vi "Calib_Analyse_fit.vi"(0 "Calib file":path, 1 "Input points":dbl[][](array[numeric]) format="%.2f", 2 "polynomial order":i32=2, 5 "Fixed n":bool=TRUE, 7 "n":dbl=0.45 format="%.2f", 9 "Point selector 3":cluster{"Y":dbl, "X":dbl, "t/f":bool}[](array[cluster]) {"X" format="%.2f"; "Y" format="%.2f"}, 11 "Point selector 4":T1(array[cluster])=[{"Y"=3.5155385742, "Y2"=3.2773117676, "X"=-15.0, "t/f"=FALSE}, {"Y"=3.4946367187, "Y2"=3.3075422363, "X"=-10.0, "t/f"=FALSE}, {"Y"=3.473232666, "Y2"=3.3353713379, "X"=-5.0, "t/f"=FALSE}, {"Y"=3.454592041, "Y2"=3.3658986816, "X"=0.0, "t/f"=FALSE}, {"Y"=3.4246572266, "Y2"=3.3874455566, "X"=5.0, "t/f"=FALSE}, {"Y"=3.398965332, "Y2"=3.4137351074, "X"=10.0, "t/f"=FALSE}, {"Y"=3.362712646484375, "Y2"=3.428485595703125, "X"=15.0, "t/f"=FALSE}] {"Y2" format="%.2f"; "X" format="%.2f"; "Y" format="%.2f"}) -> (4 "Calib const":string[][](array[string])=[["n", "0.405000"], ["A", "7.730378"], ["B", "6.204067"], ["Av % err", "0.204301"]], 6 "Calibration plot":cluster{cluster{dbl, dbl}[]}[](graph)=[{[{0.8450215822560672, 12.972948762710196}, {0.9063644870167936, 13.35352428024258}, {1.0129933166229186, 14.015056729178777}, {1.0924501688964157, 14.50801239851709}, {1.2215481063301497, 15.308944707524116}, {1.3521910897315237, 16.119462585897956}, {1.4772434835777744, 16.895296069694275}]}, {[{0.8450215822560672, 12.97084622363197}, {0.9063644870167936, 13.353228276297402}, {1.0129933166229186, 14.026771757587431}, {1.0924501688964157, 14.499243467101884}, {1.2215481063301497, 15.307992219000921}, {1.3521910897315237, 16.116882250583185}, {1.4772434835777744, 16.898281339562185}]}], 8 "Average Temp":dbl=19.0 format="%.2f", 10 "Point selector 3 out":cluster{"Y":dbl, "X":dbl, "t/f":bool}[](array[cluster]) {"X" format="%.2f"; "Y" format="%.2f"}, 14 "Coefficients":dbl[][](array[numeric]) format="%.2f", 15 "Point selector 4 out":T1(array[cluster])=[{"Y"=3.5155385742, "Y2"=3.2773117676, "X"=-15.0, "t/f"=FALSE}, {"Y"=3.4946367187, "Y2"=3.3075422363, "X"=-10.0, "t/f"=FALSE}, {"Y"=3.473232666, "Y2"=3.3353713379, "X"=-5.0, "t/f"=FALSE}, {"Y"=3.454592041, "Y2"=3.3658986816, "X"=0.0, "t/f"=FALSE}, {"Y"=3.4246572266, "Y2"=3.3874455566, "X"=5.0, "t/f"=FALSE}, {"Y"=3.398965332, "Y2"=3.4137351074, "X"=10.0, "t/f"=FALSE}, {"Y"=3.362712646484375, "Y2"=3.428485595703125, "X"=15.0, "t/f"=FALSE}] {"Y2" format="%.2f"; "X" format="%.2f"; "Y" format="%.2f"})   [LabVIEW 2014]
uses:
  <vilib>/Analysis/baseanly.llb/Mean (DBL).vi
  Globals/Calib_global.vi
  Acquisition/PWA/PWAtasksGLOBAL.vi
  <vilib>/Analysis/NI_AALBase.lvlib
panel:
  out "GMU:Source:ppm/%Density":dbl format="%.2f"
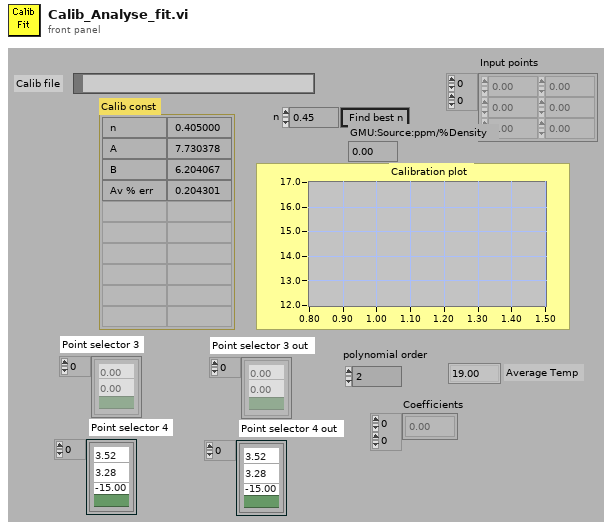
[diagram p1: front panel]
types:
  T1 = cluster{"Y":dbl, "Y2":dbl, "X":dbl, "t/f":bool}[]
  T2 = typedef "Cal_Inst_type.ctl" = enum16{"Propeller anemometer", "Pressure Transducer", "Hot wire", "Cross wire velocity", "Cross wire angle", "Generic Linear", "Generic Polynomial", "Generic BackPoly", "Fast FID", "Thermocouple", "Cold wire", "Pulsed Wire"}
  T3 = cluster{"Y":dbl, "Y":dbl, "X":dbl, "switch":bool}
  T4 = typedef "Ref_Inst_type.ctl" = enum16{"Propellor anemometer", "Pressure Transducer", "Raw voltage", "Pitot-static tube", "Preston tube", "Generic Linear", "Generic Polynomial", "Thermocouple", "LDA", "Enter Value", "ADAM Channel"}
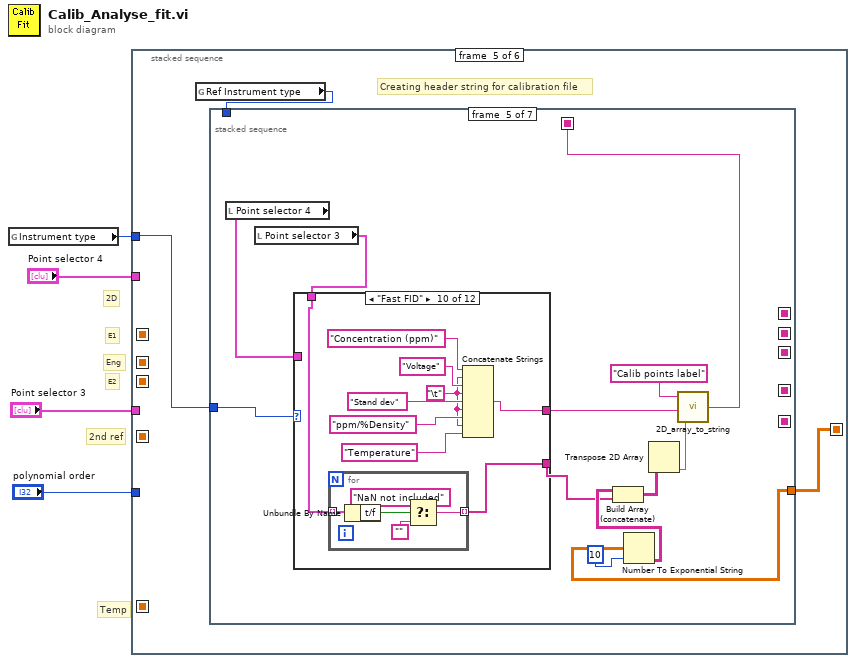
[diagram p0: block diagram]
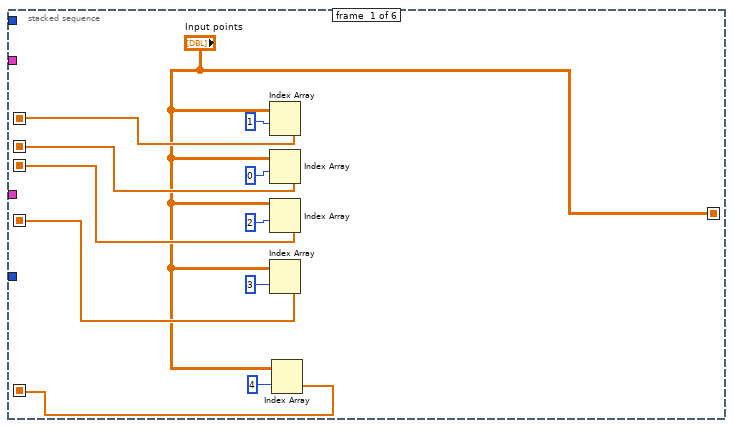
[diagram p2: hidden frame]
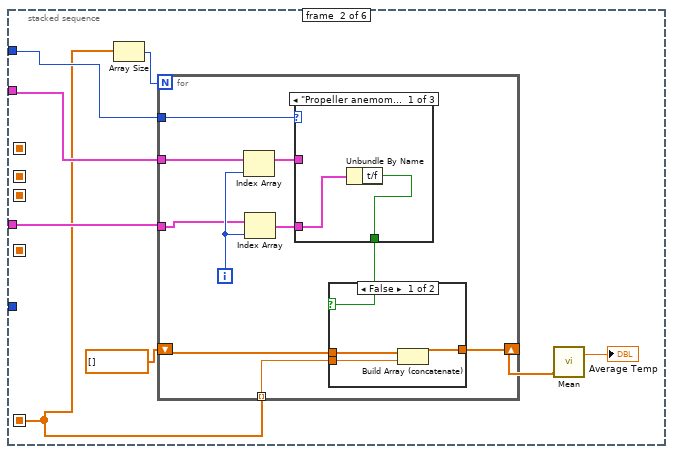
[diagram p3: hidden frame]
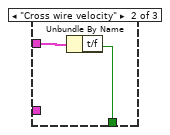
[diagram p5: hidden frame]
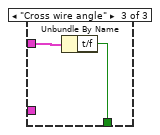
[diagram p6: hidden frame]
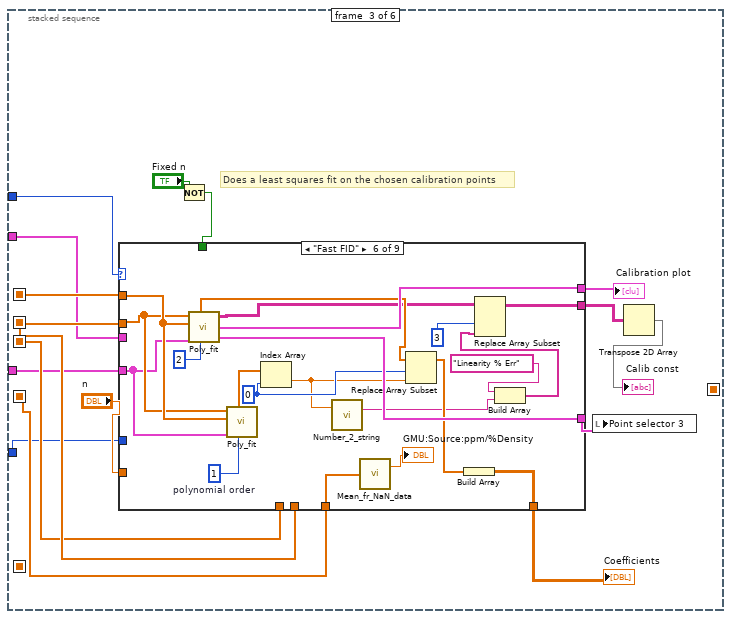
[diagram p7: hidden frame]
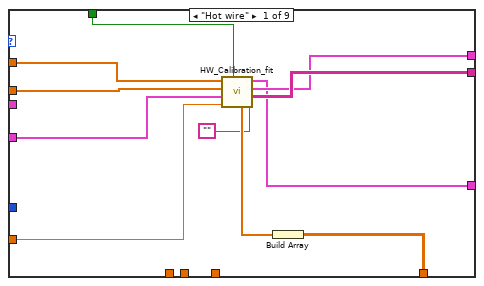
[diagram p8: hidden frame]
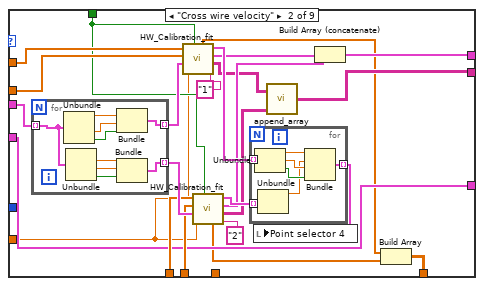
[diagram p9: hidden frame]
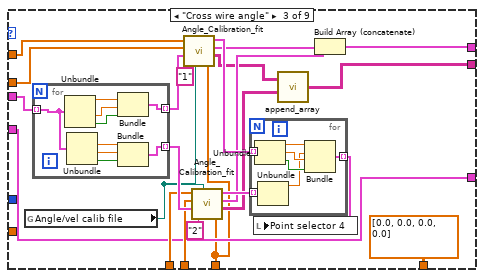
[diagram p10: hidden frame]
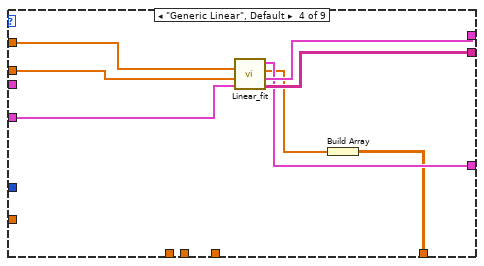
[diagram p11: hidden frame]
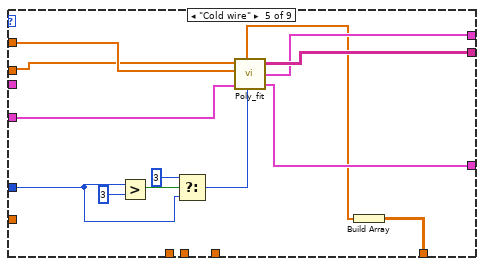
[diagram p12: hidden frame]
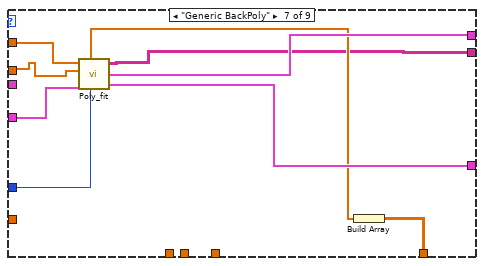
[diagram p13: hidden frame]
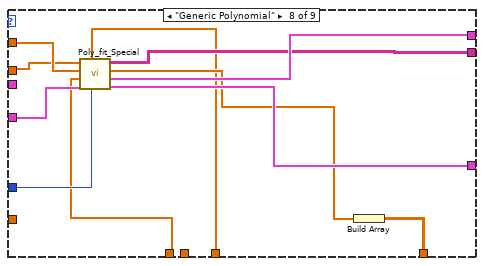
[diagram p14: hidden frame]
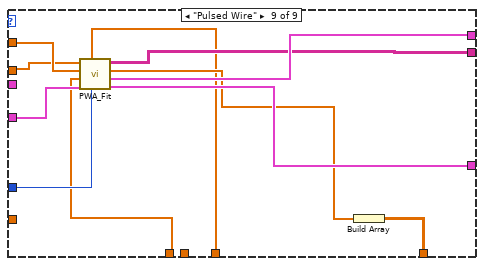
[diagram p15: hidden frame]
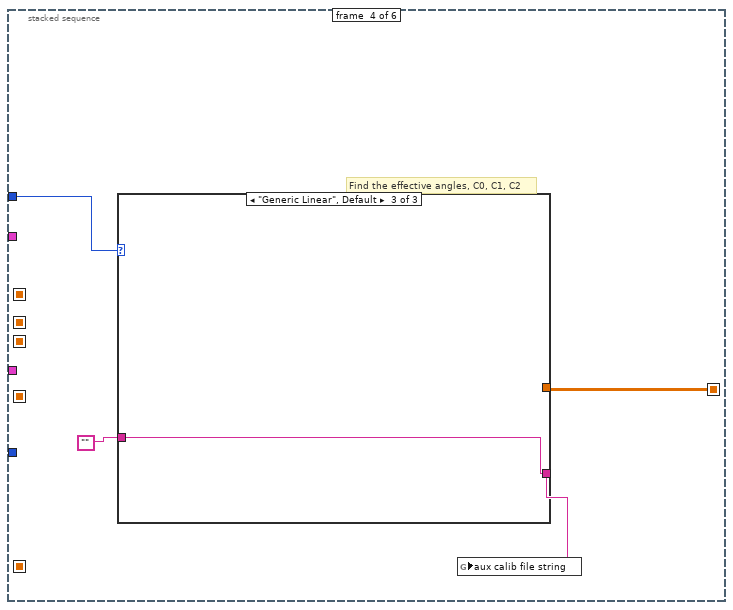
[diagram p16: hidden frame]
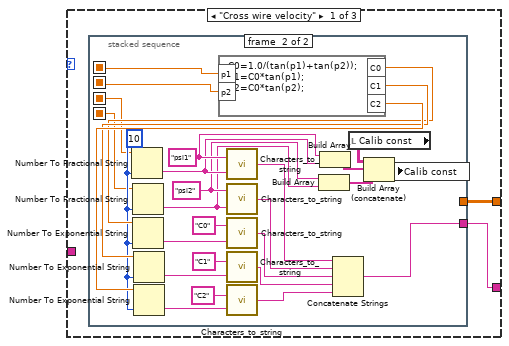
[diagram p17: hidden frame]
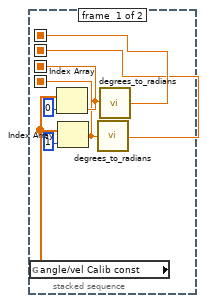
[diagram p18: hidden frame]
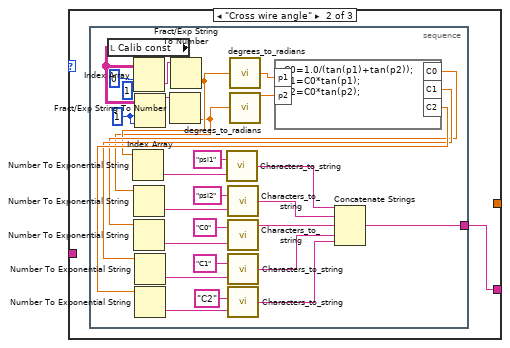
[diagram p19: hidden frame]
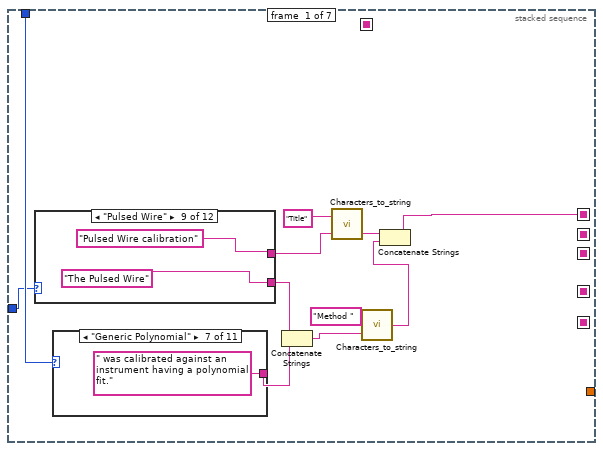
[diagram p20: hidden frame]
diagram:
  # "Temp"
  # "2D"
  # "2nd ref"
  # "E2"
  # "E1"
  # "Eng"
  n1 = global read "Calib_global.vi" "Instrument type"() -> (w4:T2)
  n2 = stacked-sequence {
    seq-local: ["Input points" _ _ _ _ _] -> [_ _ _ w223 w295 _]
    seq-local: [w11 _ _ _ _ _] -> [_ _ w52 _ _ _]
    seq-local: [w10 _ _ _ _ _] -> [_ _ w51 _ _ _]
    seq-local: [w9 _ _ _ _ _] -> [_ _ w50 _ _ _]
    seq-local: [w8 _ _ _ _ _] -> [_ _ w49 _ _ _]
    seq-local: [w5 _ _ _ _ _] -> [_ w17 _ _ _ _]
    tunnel: w4 -> [_ w23 w46 w222 w294 _]
    tunnel: "Point selector 3" -> [_ w22 w48 _ _ _]
    tunnel: "Point selector 4" -> [_ w21 w47 _ _ _]
    tunnel: "polynomial order" -> [_ _ w44 _ _ _]
    frame #0 {
      n3 = Index Array(array="Input points", index (row)=1) -> (element=w11:dbl[])  [unwired: 1 in]
      n4 = Index Array(array="Input points", index (row)=0) -> (element=w10:dbl[])  [unwired: 1 in]
      n5 = Index Array(array="Input points", index (row)=2) -> (element=w9:dbl[])  [unwired: 1 in]
      n6 = Index Array(array="Input points", index (row)=3) -> (element=w8:dbl[])  [unwired: 1 in]
      n7 = Index Array(array="Input points", index (row)=4) -> (element=w5:dbl[])  [unwired: 1 in]
    }
    frame #1 {
      n8 = Array Size(array=w17) -> (size(s)=w16:i32)
      n9 = for {
        N: w16 -> [_]
        tunnel: w23 -> [w33]
        tunnel: w22 -> [w25]
        tunnel: w21 -> [w27]
        shift-right: [w30] -> w18
        shift-left: dbl[] [] -> [w31]
        tunnel: w17 -> [w29] mode=indexing
        i -> [w26]
        n10 = Index Array(array=w27, index=w26) -> (element=w28:cluster{"Y":dbl, "Y2":dbl, "X":dbl, "t/f":bool})
        n11 = Index Array(array=w25, index=w26) -> (element=w24:cluster{"Y":dbl, "X":dbl, "t/f":bool})
        n12 = case shown="\"Propeller anemometer\", Default" w33 {
          tunnel: w24 -> [w39 _ _]
          tunnel: w28 -> [_ w41 w43]
          tunnel: [w38 w40 w42] -> w32
          frame "Propeller anemometer", Default {
            n13 = Unbundle By Name(w39) -> ("t/f"=w38:bool)
          }
          frame "Cross wire velocity" {
            n14 = Unbundle By Name(w41) -> ("t/f"=w40:bool)
          }
          frame "Cross wire angle" {
            n15 = Unbundle By Name(w43) -> ("t/f"=w42:bool)
          }
        }
        n16 = case shown="False" w32 {
          tunnel: w31 -> [w36 w37]
          tunnel: [w35 w37] -> w30
          tunnel: w29 -> [w34 _]
          frame False {
            n17 = Build Array (concatenate)(w36, w34) -> (w35:dbl[])
          }
          frame True {
          }
        }
      }
      n18 = call-poly <vilib>:"Mean.vi"("X"=w18) -> ("mean"=→"Average Temp":dbl)  [unwired: 1 out]
    }
    frame #2 {
      # "Does a least squares fit on the chosen calibration points"
      n19 = Not(x="Fixed n") -> (.not. x?=w54:bool)
      n20 = case shown="\"Fast FID\"" w46 {
        tunnel: [w65 w82 w120 w151 w166 w189 w198 w209 w220] -> w57
        tunnel: w52 -> [w70 w94 w132 w156 w165 w178 w195 w207 w218]
        tunnel: w51 -> [w69 w93 w131 w155 w164 w177 w194 w206 w217]
        tunnel: w54 -> [w68 w80 _ _ _ _ _ _ _]
        tunnel: w47 -> [_ w83 w121 _ _ _ _ _ _]
        tunnel: [w67 w76 w114 w154 w169 w179 w192 w203 w214] -> w55
        tunnel: [w66 w84 w122 w153 w168 w190 w199 w210 w221] -> w56
        tunnel: w51 -> [_ w89 w127 _ _ _ _ _ _]
        tunnel: w50 -> [_ w88 w126 _ _ _ _ w201 w212]
        tunnel: w48 -> [w64 w82 w120 w152 w167 w176 w196 w205 w216]
        tunnel: "n" -> [w63 w79 _ _ _ _ _ _ _]
        tunnel: w49 -> [_ _ w113 _ _ w171 _ w200 w211]
        tunnel: [w61 w73 dbl[][] [[0.0, 0.0], [0.0, 0.0]] w149 w158 w188 w197 w208 w219] -> w45
        tunnel: w44 -> [_ _ _ _ w157 _ w191 w202 w213]
        frame "Hot wire" {
          n21 = call "HW_Calibration_fit.vi"("coeff suffix"="", "Fixed n (F)"=w68, "n input  (0.45)"=w63, "Point selector"=w64, "Velocity"=w69, "HW voltage"=w70) -> ("Calib const"=w67:string[][], "Calibration plot"=w66:cluster{cluster{dbl, "mse":dbl}[]}[], "Point selector"=w65:cluster{"Y":dbl, "X":dbl, "switch":bool}[], "Coefficients"=w62:dbl[])
          n22 = Build Array(w62) -> (w61:dbl[][])
        }
        frame "Cross wire velocity" {
          n23 = for {
            tunnel: w83 -> [w106] mode=indexing
            tunnel: [w107] -> w92 mode=indexing
            tunnel: [w105] -> w90 mode=indexing
            n24 = Unbundle(w106) -> ("Y"=w110:dbl, "X"=w109:dbl, "t/f"=w108:bool)  [unwired: 1 out]
            n25 = Unbundle(w106) -> ("Y2"=w104:dbl, "X"=w103:dbl, "t/f"=w102:bool)  [unwired: 1 out]
            n26 = Bundle("Y"=w110, "X"=w109, "t/f"=w108) -> (w107:cluster{"Y":dbl, "X":dbl, "t/f":bool})  [unwired: 1 out]
            n27 = Bundle("Y2"=w104, "X"=w103, "t/f"=w102) -> (w105:cluster{"Y2":dbl, "X":dbl, "t/f":bool})  [unwired: 1 out]
          }
          n28 = call "HW_Calibration_fit.vi"("coeff suffix"="1", "Fixed n (F)"=w80, "n input  (0.45)"=w79, "Point selector"=w92, "Velocity"=w93, "HW voltage"=w94) -> ("Calib const"=w77:string[][], "Calibration plot"=w85:cluster{cluster{dbl, "mse":dbl}[]}[], "Point selector"=w91:cluster{"Y":dbl, "X":dbl, "switch":bool}[], "Coefficients"=w71:dbl[])
          n29 = call "HW_Calibration_fit.vi"("coeff suffix"="2", "Fixed n (F)"=w80, "n input  (0.45)"=w79, "Point selector"=w90, "Velocity"=w89, "HW voltage"=w88) -> ("Calib const"=w78:string[][], "Calibration plot"=w86:cluster{cluster{dbl, "mse":dbl}[]}[], "Point selector"=w87:cluster{"Y":dbl, "X":dbl, "switch":bool}[], "Coefficients"=w72:dbl[])
          n30 = for {
            tunnel: w91 -> [w101] mode=indexing
            tunnel: [w97] -> w81 mode=indexing
            tunnel: w87 -> [w96] mode=indexing
            n31 = Unbundle(w101) -> ("Y"=w100:dbl, "X"=w99:dbl, "switch"=w98:bool)
            n32 = Unbundle(w96) -> ("Y"=w95:dbl)  [unwired: 2 out]
            n33 = Bundle("Y"=w100, "Y"=w95, "X"=w99, "switch"=w98) -> (w97:T3)  [unwired: 1 out]
          }
          n34 = local write "Point selector 4"(w81) -> ()
          n35 = call "append_array.vi"("array 2"=w78, "array 1"=w77) -> ("appended array"=w76:string[][])
          n36 = Build Array (concatenate)(w85, w86) -> (w84:cluster{cluster{dbl, "mse":dbl}[]}[])
          n37 = Build Array(w71, w72) -> (w73:dbl[][])
        }
        frame "Cross wire angle" {
          n38 = global read "Calib_global.vi" "Angle/vel calib file"() -> (w112:path)
          n39 = for {
            tunnel: w121 -> [w144] mode=indexing
            tunnel: [w145] -> w130 mode=indexing
            tunnel: [w143] -> w128 mode=indexing
            n40 = Unbundle(w144) -> ("Y"=w148:dbl, "X"=w147:dbl, "t/f"=w146:bool)  [unwired: 1 out]
            n41 = Unbundle(w144) -> ("Y2"=w142:dbl, "X"=w141:dbl, "t/f"=w140:bool)  [unwired: 1 out]
            n42 = Bundle("Y"=w148, "X"=w147, "t/f"=w146) -> (w145:cluster{"Y":dbl, "X":dbl, "t/f":bool})  [unwired: 1 out]
            n43 = Bundle("Y2"=w142, "X"=w141, "t/f"=w140) -> (w143:cluster{"Y2":dbl, "X":dbl, "t/f":bool})  [unwired: 1 out]
          }
          n44 = call "Angle_Calibration_fit.vi"("Reference Velocity"=w113, "Vel calib file"=w112, "coeff suffix"="1", "Point selector"=w130, "Angle"=w131, "HW voltage"=w132) -> ("Calib const"=w116:string[][], "Angle calibration (output)"=w123:cluster{cluster{"Y":dbl, "Y":dbl}[]}[], "Point selector"=w129:cluster{"Y":dbl, "X":dbl, "switch":bool}[])
          n45 = call "Angle_Calibration_fit.vi"("Reference Velocity"=w113, "Vel calib file"=w112, "coeff suffix"="2", "Point selector"=w128, "Angle"=w127, "HW voltage"=w126) -> ("Calib const"=w115:string[][], "Angle calibration (output)"=w124:cluster{cluster{"Y":dbl, "Y":dbl}[]}[], "Point selector"=w125:cluster{"Y":dbl, "X":dbl, "switch":bool}[])
          n46 = for {
            tunnel: w129 -> [w139] mode=indexing
            tunnel: [w135] -> w119 mode=indexing
            tunnel: w125 -> [w134] mode=indexing
            n47 = Unbundle(w139) -> ("Y"=w138:dbl, "X"=w137:dbl, "switch"=w136:bool)
            n48 = Unbundle(w134) -> ("Y"=w133:dbl)  [unwired: 2 out]
            n49 = Bundle("Y"=w138, "Y"=w133, "X"=w137, "switch"=w136) -> (w135:T3)  [unwired: 1 out]
          }
          n50 = local write "Point selector 4"(w119) -> ()
          n51 = call "append_array.vi"("array 2"=w115, "array 1"=w116) -> ("appended array"=w114:string[][])
          n52 = Build Array (concatenate)(w123, w124) -> (w122:cluster{cluster{"Y":dbl, "Y":dbl}[]}[])
        }
        frame "Generic Linear", Default {
          n53 = call "Linear_fit.vi"("Point selector"=w152, "Input X array"=w155, "Input Y array"=w156) -> ("Calib const"=w154:string[][], "Calibration plot"=w153:cluster{cluster{dbl, dbl}[]}[], "Coefficients"=w150:dbl[], "Point selector"=w151:cluster{"Y":dbl, "X":dbl, "switch":bool}[])  [unwired: 1 out]
          n54 = Build Array(w150) -> (w149:dbl[][])
        }
        frame "Cold wire" {
          n55 = Greater?(x=w157, y=3) -> (0:w162:bool)
          n56 = Select(t=3, s=w162, f=w157) -> (s? t:f=w160:i32)
          n57 = call "Poly_fit.vi"("Input Y array"=w164, "Input X array"=w165, "polynomial order"=w160, "Point selector"=w167) -> ("Coefficients"=w159:dbl[], "Calib const"=w169:string[][], "Calibration plot"=w168:cluster{cluster{dbl, dbl}[]}[], "Point selector"=w166:cluster{"Y":dbl, "X":dbl, "switch":bool}[])  [unwired: 1 out]
          n58 = Build Array(w159) -> (w158:dbl[][])
        }
        frame "Fast FID" {
          w183 = 0 ("index")
          w186 = 1  # polynomial order
          n59 = call "Poly_fit.vi"("Input Y array"=w177, "Input X array"=w178, "polynomial order"=2, "Point selector"=w176) -> ("Coefficients"=w184:dbl[], "Calib const"=w181:string[][], "Calibration plot"=w190:cluster{cluster{dbl, dbl}[]}[], "Point selector"=w189:cluster{"Y":dbl, "X":dbl, "switch":bool}[])  [unwired: 1 out]
          n60 = call "Poly_fit.vi"("Input Y array"=w177, "Input X array"=w178, "polynomial order"=w186, "Point selector"=w176) -> ("Coefficients"=w185:dbl[])  [unwired: 4 out]
          n61 = Index Array(array=w185, index=w183) -> (element=w175:dbl)
          n62 = call "Number_2_string.vi"("number"=w175) -> ("String"=w173:string)  [unwired: 1 in]
          n63 = call "Mean_fr_NaN_data.vi"("Data"=w171) -> ("Mean value"=→"GMU:Source:ppm/%Density":dbl)  [unwired: 1 out]
          n64 = Replace Array Subset(array=w184, new element=w175, index=w183) -> (w182:dbl[])
          n65 = Build Array(w182) -> (w188:dbl[][])
          n66 = Build Array("Linearity % Err" ("new element/subarray"), w173) -> (w172:string[])
          n67 = Replace Array Subset(array=w181, new element=w172, index (col)=3 ("disabled index (col)")) -> (w179:string[][])  [unwired: 1 in]
        }
        frame "Generic BackPoly" {
          n68 = call "Poly_fit.vi"("Input Y array"=w195, "Input X array"=w194, "polynomial order"=w191, "Point selector"=w196) -> ("Coefficients"=w193:dbl[], "Calib const"=w192:string[][], "Calibration plot"=w199:cluster{cluster{dbl, dbl}[]}[], "Point selector"=w198:cluster{"Y":dbl, "X":dbl, "switch":bool}[])  [unwired: 1 out]
          n69 = Build Array(w193) -> (w197:dbl[][])
        }
        frame "Generic Polynomial" {
          n70 = call "Poly_fit_Special.vi"("polynomial order"=w202, "Input X^3"=w200, "Point selector"=w205, "Input X^2"=w201, "Input X array"=w207, "Input Y array"=w206) -> ("Point selector"=w209:cluster{"Y":dbl, "X":dbl, "switch":bool}[], "Calibration plot"=w210:cluster{cluster{dbl, dbl}[]}[], "Coefficients"=w204:dbl[], "Calib const"=w203:string[][])
          n71 = Build Array(w204) -> (w208:dbl[][])
        }
        frame "Pulsed Wire" {
          n72 = call "PWA_Fit.vi"("polynomial order"=w213, "Input X^3"=w211, "Point selector"=w216, "Input X^2"=w212, "Input X array"=w218, "Input Y array"=w217) -> ("Point selector"=w220:cluster{"Y":dbl, "X":dbl, "switch":bool}[], "Calibration plot"=w221:cluster{cluster{dbl, dbl}[]}[], "Coefficients"=w215:dbl[], "Calib const"=w214:string[][])
          n73 = Build Array(w215) -> (w219:dbl[][])
        }
      }
      "Calibration plot" <- w56
      "Coefficients" <- w45
      n74 = local write "Point selector 3"(w57) -> ()
      n75 = Transpose 2D Array(2D array=w55) -> (transposed array=→"Calib const":string[][])
    }
    frame #3 {
      # "Find the effective angles, C0, C1, C2"
      n76 = case shown="\"Generic Linear\", Default" w222 {
        tunnel: "" -> [_ _ w293]
        tunnel: [w227 w263 w293] -> w225
        tunnel: w223 -> [w226 _ _]
        frame "Cross wire velocity" {
          n77 = stacked-sequence {
            seq-local: [w232 _] -> [_ w238]
            seq-local: [w231 _] -> [_ w236]
            seq-local: [w230 _] -> [_ w237]
            seq-local: [w229 _] -> [_ w235]
            tunnel: [_ w248] -> w227
            tunnel: w226 -> [_ _]
            frame #0 {
              n78 = global read "Calib_global.vi" "angle/vel Calib const"() -> (w228:dbl[])
              n79 = Index Array(array=w228, index=0) -> (element=w230:dbl)
              n80 = Index Array(array=w228, index=1) -> (element=w229:dbl)
              n81 = call "degrees_to_radians.vi"("degrees"=w229) -> ("radians"=w231:dbl)
              n82 = call "degrees_to_radians.vi"("degrees"=w230) -> ("radians"=w232:dbl)
            }
            frame #1 {
              w239 = 10
              w245 = "psi2"
              w247 = "psi1"
              n83 = Number To Fractional String(number=w237, precision (6)=w239) -> (F-format string=w246:string)  [unwired: 2 out]
              n84 = Number To Fractional String(number=w235, precision (6)=w239) -> (F-format string=w244:string)  [unwired: 2 out]
              n85 = formula code="C0=1.0/(tan(p1)+tan(p2));\nC1=C0*tan(p1);\nC2=C0*tan(p2);"("p1"=w238, "p2"=w236) -> ("C0"=w260:dbl, "C1"=w261:dbl, "C2"=w262:dbl)
              n86 = Number To Exponential String(number=w260, precision (6)=w239) -> (E-format string=w258:string)  [unwired: 2 out]
              n87 = Number To Exponential String(number=w261, precision (6)=w239) -> (E-format string=w256:string)  [unwired: 2 out]
              n88 = Number To Exponential String(number=w262, precision (6)=w239) -> (E-format string=w254:string)  [unwired: 2 out]
              n89 = call "Characters_to_string.vi"("Characters to write"=w246, "Label for characters"=w247) -> ("Output string"=w252:string)
              n90 = call "Characters_to_string.vi"("Characters to write"=w244, "Label for characters"=w245) -> ("Output string"=w251:string)
              n91 = call "Characters_to_string.vi"("Characters to write"=w258, "Label for characters"="C0") -> ("Output string"=w253:string)
              n92 = call "Characters_to_string.vi"("Characters to write"=w256, "Label for characters"="C1") -> ("Output string"=w250:string)
              n93 = call "Characters_to_string.vi"("Characters to write"=w254, "Label for characters"="C2") -> ("Output string"=w249:string)
              n94 = Build Array(w245, w244) -> (w242:string[])
              n95 = Build Array(w247, w246) -> (w243:string[])
              n96 = Concatenate Strings(w252, w251, w253, w250, w249) -> (w248:string)
              n97 = local read "Calib const"() -> (w241:string[][])
              n98 = Build Array (concatenate)(w241, w243, w242) -> (w240:string[][])
              n99 = local write "Calib const"(w240) -> ()
            }
          }
        }
        frame "Cross wire angle" {
          n100 = stacked-sequence {
            tunnel: [w274] -> w263
            frame #0 {
              w273 = 1
              n101 = local read "Calib const"() -> (w271:string[][])
              n102 = Index Array(array=w271, index (row)=0, index (col)=1) -> (element=w270:string)
              n103 = Index Array(array=w271, index (row)=w273, index (col)=w273) -> (element=w269:string)
              n104 = Fract/Exp String To Number(string=w269) -> (number=w264:dbl)  [unwired: 4 out]
              n105 = Number To Exponential String(number=w264) -> (E-format string=w286:string)  [unwired: 3 out]
              n106 = Fract/Exp String To Number(string=w270) -> (number=w267:dbl)  [unwired: 4 out]
              n107 = Number To Exponential String(number=w267) -> (E-format string=w287:string)  [unwired: 3 out]
              n108 = call "Characters_to_string.vi"("Characters to write"=w287, "Label for characters"="psi1") -> ("Output string"=w278:string)
              n109 = call "Characters_to_string.vi"("Characters to write"=w286, "Label for characters"="psi2") -> ("Output string"=w277:string)
              n110 = call "degrees_to_radians.vi"("degrees"=w267) -> ("radians"=w266:dbl)
              n111 = call "degrees_to_radians.vi"("degrees"=w264) -> ("radians"=w265:dbl)
              n112 = formula code="C0=1.0/(tan(p1)+tan(p2));\nC1=C0*tan(p1);\nC2=C0*tan(p2);"("p1"=w266, "p2"=w265) -> ("C0"=w290:dbl, "C1"=w291:dbl, "C2"=w292:dbl)
              n113 = Number To Exponential String(number=w290) -> (E-format string=w284:string)  [unwired: 3 out]
              n114 = Number To Exponential String(number=w291) -> (E-format string=w282:string)  [unwired: 3 out]
              n115 = Number To Exponential String(number=w292) -> (E-format string=w280:string)  [unwired: 3 out]
              n116 = call "Characters_to_string.vi"("Characters to write"=w284, "Label for characters"="C0") -> ("Output string"=w279:string)
              n117 = call "Characters_to_string.vi"("Characters to write"=w282, "Label for characters"="C1") -> ("Output string"=w276:string)
              n118 = call "Characters_to_string.vi"("Characters to write"=w280, "Label for characters"="C2") -> ("Output string"=w275:string)
              n119 = Concatenate Strings(w278, w277, w279, w276, w275) -> (w274:string)
            }
          }
        }
        frame "Generic Linear", Default {
        }
      }
      n120 = global write "Calib_global.vi" "aux calib file string"(w225) -> ()
    }
    frame #4 {
      # "Creating header string for calibration file"
      n121 = global read "Calib_global.vi" "Ref Instrument type"() -> (w296:T4)
      n122 = stacked-sequence {
        seq-local: [_ w357 _ _ _ _ _] -> [_ _ _ _ _ _ w657]
        seq-local: [w305 _ _ _ _ _ _] -> [_ _ _ _ _ _ w658]
        seq-local: [_ _ w369 _ _ _ _] -> [_ _ _ _ _ _ w656]
        seq-local: [_ _ _ w383 _ _ _] -> [_ _ _ _ _ _ w653]
        seq-local: [_ _ _ _ _ w636 _] -> [_ _ _ _ _ _ w654]
        seq-local: [_ _ _ _ w488 _ _] -> [_ _ _ _ _ w637 _]
        tunnel: w296 -> [w300 _ _ _ _ _ _]
        tunnel: w295 -> [_ _ _ _ w485 _ _]
        tunnel: w294 -> [w297 w350 _ w381 w479 w635 w659]
        frame #0 {
          n123 = case shown="\"Pulsed Wire\"" w297 {
            tunnel: ["Propeller Anemometer velocity calibration" "Pressure Transducer calibration" "Hot wire velocity calibration" "Cross wire velocity calibration" "Cross wire angle calibration" "Fast FID calibration" "Generic Linear calibration" "Generic Polynomial calibration" "Pulsed Wire calibration" "Generic Backwards Polynomial calibration" "Thermocouple calibration" "Cold wire calibration"] -> w304
            tunnel: ["The Propeller Anemometer" "The Pressure Transducer" "The Hot wire" "The Cross wire" "The Cross wire" "The Fast FID" "The Generic Linear Instrument" "The Generic Polynomial Instrument" "The Pulsed Wire" "The Generic Backwards Polynomial Instrument" "The Thermocouple" "The Cold wire"] -> w301
            frame "Propeller anemometer" {
            }
            frame "Pressure Transducer" {
            }
            frame "Hot wire" {
            }
            frame "Cross wire velocity" {
            }
            frame "Cross wire angle" {
            }
            frame "Fast FID" {
            }
            frame "Generic Linear" {
            }
            frame "Generic Polynomial" {
            }
            frame "Pulsed Wire" {
            }
            frame "Generic BackPoly" {
            }
            frame "Thermocouple" {
            }
            frame "Cold wire" {
            }
          }
          n124 = case shown="\"Generic Polynomial\"" w300 {
            tunnel: [" was calibrated for velocity against a Propeller Anemometer." " was calibrated for pressure against a Pressure Transducer." " was calibrated against a voltage" " was calibrated for velocity against a Pitot-static tube." " was calibrated against a Preston tube." " was calibrated against an instrument having a Linear fit." " was calibrated against an instrument having a polynomial fit." " was calibrated for temperature against a thermocouple." " was calibrated for velocity against the LDA." " was calibrated against the reading entered by the user." " was calibrated against an ADAM channel."] -> w302
            frame "Propellor anemometer" {
            }
            frame "Pressure Transducer" {
            }
            frame "Raw voltage" {
            }
            frame "Pitot-static tube" {
            }
            frame "Preston tube" {
            }
            frame "Generic Linear" {
            }
            frame "Generic Polynomial" {
            }
            frame "Thermocouple" {
            }
            frame "LDA" {
            }
            frame "Enter Value" {
            }
            frame "ADAM Channel" {
            }
          }
          n125 = Concatenate Strings(w301, w302) -> (w299:string)
          n126 = call "Characters_to_string.vi"("Characters to write"=w304, "Label for characters"="Title") -> ("Output string"=w306:string)
          n127 = call "Characters_to_string.vi"("Characters to write"=w299, "Label for characters"="Method ") -> ("Output string"=w298:string)
          n128 = Concatenate Strings(w306, w298) -> (w305:string)
        }
        frame #1 {
          n129 = local read "Average Temp"() -> (w349:dbl)
          n130 = case shown="\"Fast FID\"" w350 {
            tunnel: [w362 "" w367] -> w353
            frame "Cross wire angle" {
              n131 = global read "Calib_global.vi" "Angle/vel calib file"() -> (w361:path)
              n132 = Strip Path(path=w361) -> (name=w360:string)  [unwired: 1 out]
              n133 = call "Characters_to_string.vi"("Characters to write"=w360, "Label for characters"="Original vel calib") -> ("Output string"=w362:string)
            }
            frame "Generic Linear", Default {
            }
            frame "Fast FID" {
              n134 = local read "GMU:Source:ppm/%Density"() -> (w366:dbl)
              n135 = call "Value_to_string.vi"("Value"=w366, "Label for value"="GMU:Source:ppm/%Density") -> ("Output string"=w367:string)  [unwired: 1 in]
            }
          }
          n136 = global read "Calib_global.vi" "Abs Press (mbar)"() -> (w352:dbl)
          n137 = Strip Path(path="Calib file") -> (name=w347:string)  [unwired: 1 out]
          n138 = call "Characters_to_string.vi"("Characters to write"="Calibration_File", "Label for characters"="File_Type") -> ("Output string"=w343:string)
          n139 = call "Value_to_string.vi"("Value"=w349, "Label for value"="Calib temp") -> ("Output string"=w354:string)  [unwired: 1 in]
          n140 = call "Value_to_string.vi"("Value"=w352, "Label for value"="Abs Press (mbar)") -> ("Output string"=w355:string)  [unwired: 1 in]
          n141 = call "Characters_to_string.vi"("Characters to write"=w347, "Label for characters"="File name") -> ("Output string"=w344:string)
          n142 = call "Date_and_Time_to_string.vi"() -> ("Date and time (spreadsheet)"=w356:string)
          n143 = Concatenate Strings(w356, w344, w343, w353, w354, w355) -> (w357:string)
        }
        frame #2 {
          n144 = global read "Calib_global.vi" "Ref Inst present"() -> (w368:bool)
          n145 = case shown="True" w368 {
            tunnel: ["" w376] -> w369
            frame False {
            }
            frame True {
              n146 = global read "Calib_global.vi" "Ref Calib file"() -> (w372:path)
              n147 = Strip Path(path=w372) -> (name=w371:string)  [unwired: 1 out]
              n148 = Concatenate Strings("Ref Inst calib file", "\t", w371, "\r\n") -> (w376:string)
            }
          }
        }
        frame #3 {
          n149 = local read "Calib const"() -> (w377:string[][])
          n150 = Index Array(array=w377, index (col)=1) -> (element=w379:string[])  [unwired: 1 in]
          n151 = case shown="\"Pulsed Wire\"" w381 {
            tunnel: [w398 w411 w416 w425 w438 w449 w461 w467 w478] -> w382
            tunnel: w379 -> [_ _ w419 w428 w441 w452 _ _ _]
            tunnel: [2 ("Index") 3 ("Index") 6 ("Index") 9 ("Index") 6 ("Index") 4 ("Index") 3 ("Index") 2 ("Index") 7 ("Index")] -> w380
            tunnel: ["Av % Err" "Linearity % Err" "Av % Err" "Av % err -ve" "Av % Err" "Av % Err" "Av % Err" "Av % Err" "Av % Err"] -> w378
            tunnel: w377 -> [_ _ _ w430 _ _ _ _ _]
            frame "Propeller anemometer", Default {
              n152 = Build Array("Coeff A", "Coeff B") -> (w398:string[])
            }
            frame "Fast FID" {
              n153 = Build Array("Coeff A", "Coeff B", "Coeff C", "Fast FID Bkgnd", "Fast FID Bkgnd Variance", "FFID Bkgnd Volts", "FFID Bkgnd Time", "FFID Bkgnd Filename") -> (w411:string[])
            }
            frame "Generic Polynomial" {
              n154 = Array Size(array=w419) -> (size(s)=w420:i32)
              n155 = Decrement(x=w420) -> (x-1=w418:i32)
              n156 = Build Array("Coeff A", "Coeff B", "Coeff C", "Coeff D", "Coeff E", "Coeff F") -> (w417:string[])
              n157 = Array Subset(array=w417, length=w418) -> (w416:string[])  [unwired: 1 in]
            }
            frame "Pulsed Wire" {
              n158 = Array Size(array=w428) -> (size(s)=w429:i32)
              n159 = Index Array(array=w430, index (col)=0) -> (element=w427:string[])  [unwired: 1 in]
              n160 = Decrement(x=w429) -> (x-1=w426:i32)
              n161 = Array Subset(array=w427, length=w426) -> (w425:string[])  [unwired: 1 in]
            }
            frame "Generic BackPoly" {
              n162 = Array Size(array=w441) -> (size(s)=w442:i32)
              n163 = Decrement(x=w442) -> (x-1=w440:i32)
              n164 = Build Array("Coeff A", "Coeff B", "Coeff C", "Coeff D", "Coeff E", "Coeff F") -> (w439:string[])
              n165 = Array Subset(array=w439, length=w440) -> (w438:string[])  [unwired: 1 in]
            }
            frame "Cold wire" {
              n166 = Array Size(array=w452) -> (size(s)=w453:i32)
              n167 = Decrement(x=w453) -> (x-1=w451:i32)
              n168 = Build Array("Coeff A", "Coeff B", "Coeff C", "Coeff D") -> (w450:string[])
              n169 = Array Subset(array=w450, length=w451) -> (w449:string[])  [unwired: 1 in]
            }
            frame "Hot wire" {
              n170 = Build Array("Coeff n", "Coeff A", "Coeff B") -> (w461:string[])
            }
            frame "Cross wire angle" {
              n171 = Build Array("psi1", "psi2") -> (w467:string[])
            }
            frame "Cross wire velocity" {
              n172 = Build Array("Coeff n1", "Coeff A1", "Coeff B1", "Av % Err", "Coeff n2", "Coeff A2", "Coeff B2") -> (w478:string[])
            }
          }
          n173 = for {
            shift-right: [w394] -> w386
            shift-left: "\r\n" -> [w395]
            tunnel: w382 -> [w393] mode=indexing
            tunnel: w379 -> [w391]
            i -> [w392]
            n174 = Index Array(array=w391, index=w392) -> (element=w390:string)
            n175 = call "Characters_to_string.vi"("Characters to write"=w390, "Label for characters"=w393) -> ("Output string"=w389:string)
            n176 = Concatenate Strings(w395, w389) -> (w394:string)
          }
          n177 = Index Array(array=w379, index=w380) -> (element=w385:string)
          n178 = call "Characters_to_string.vi"("Characters to write"=w385, "Label for characters"=w378) -> ("Output string"=w387:string)
          n179 = Concatenate Strings(w386, w387) -> (w383:string)
        }
        frame #4 {
          n180 = local read "Point selector 4"() -> (w486:T1)
          n181 = local read "Point selector 3"() -> (w487:cluster{"Y":dbl, "X":dbl, "t/f":bool}[])
          n182 = case shown="\"Fast FID\"" w479 {
            tunnel: [w493 w504 w515 w529 w542 w552 w567 w581 w591 w606 w616 w627] -> w489
            tunnel: w487 -> [w492 w503 w514 _ _ w551 w566 w580 w590 w605 w615 w626]
            tunnel: w486 -> [_ _ _ w527 w541 _ _ _ _ _ _ _]
            tunnel: [w491 w502 w513 w526 w538 w550 w565 w578 w589 w604 w614 w625] -> w483
            frame "Propeller anemometer" {
              n183 = for {
                tunnel: w492 -> [w501] mode=indexing
                tunnel: [w499] -> w491 mode=indexing
                n184 = Unbundle By Name(w501) -> ("t/f"=w500:bool)
                n185 = Select(t="NaN not included", s=w500, f="") -> (s? t:f=w499:string)
              }
              n186 = Concatenate Strings("Velocity m/s", "\t", "Voltage") -> (w493:string)
            }
            frame "Pressure Transducer" {
              n187 = for {
                tunnel: w503 -> [w510] mode=indexing
                tunnel: [w511] -> w502 mode=indexing
                n188 = Unbundle By Name(w510) -> ("t/f"=w512:bool)
                n189 = Select(t="NaN not included", s=w512, f="") -> (s? t:f=w511:string)
              }
              n190 = Concatenate Strings("Pressure mmH2O", "\t", "Voltage") -> (w504:string)
            }
            frame "Hot wire" {
              n191 = for {
                tunnel: w514 -> [w523] mode=indexing
                tunnel: [w521] -> w513 mode=indexing
                n192 = Unbundle By Name(w523) -> ("t/f"=w522:bool)
                n193 = Select(t="NaN not included", s=w522, f="") -> (s? t:f=w521:string)
              }
              n194 = Concatenate Strings("Velocity m/s", "\t", "Voltage") -> (w515:string)
            }
            frame "Cross wire velocity" {
              w528 = "\t"
              n195 = for {
                tunnel: w527 -> [w535] mode=indexing
                tunnel: [w534] -> w526 mode=indexing
                n196 = Unbundle By Name(w535) -> ("t/f"=w532:bool)
                n197 = Select(t="NaN not included", s=w532, f="") -> (s? t:f=w534:string)
              }
              n198 = Concatenate Strings("Velocity m/s", w528, "Voltage1", w528, "Voltage2") -> (w529:string)
            }
            frame "Cross wire angle" {
              w536 = "\t"
              n199 = for {
                tunnel: w541 -> [w548] mode=indexing
                tunnel: [w546] -> w538 mode=indexing
                n200 = Unbundle By Name(w548) -> ("t/f"=w547:bool)
                n201 = Select(t="NaN not included", s=w547, f="") -> (s? t:f=w546:string)
              }
              n202 = Concatenate Strings("Angle (degrees)", w536, "Voltage1", w536, "Voltage2", w536, "Ref velocity") -> (w542:string)
            }
            frame "Generic Linear" {
              n203 = global read "Calib_global.vi" "calib units"() -> (w549:string)
              n204 = for {
                tunnel: w551 -> [w559] mode=indexing
                tunnel: [w557] -> w550 mode=indexing
                n205 = Unbundle By Name(w559) -> ("t/f"=w558:bool)
                n206 = Select(t="NaN not included", s=w558, f="") -> (s? t:f=w557:string)
              }
              n207 = Concatenate Strings(w549, "\t", "Voltage") -> (w552:string)
            }
            frame "Generic Polynomial" {
              w563 = "\t"
              n208 = global read "Calib_global.vi" "calib units"() -> (w564:string)
              n209 = for {
                tunnel: w566 -> [w573] mode=indexing
                tunnel: [w571] -> w565 mode=indexing
                n210 = Unbundle By Name(w573) -> ("t/f"=w572:bool)
                n211 = Select(t="NaN not included", s=w572, f="") -> (s? t:f=w571:string)
              }
              n212 = Concatenate Strings(w564, w563, "Volts", w563, "Volts^2", w563, "Volts^3", "Temperature") -> (w567:string)
            }
            frame "Pulsed Wire" {
              w575 = "\t"
              n213 = for {
                tunnel: w580 -> [w587] mode=indexing
                tunnel: [w585] -> w578 mode=indexing
                n214 = Unbundle By Name(w587) -> ("t/f"=w586:bool)
                n215 = Select(t="NaN not included", s=w586, f="") -> (s? t:f=w585:string)
              }
              n216 = Concatenate Strings("Velocity or Tau" ("string"), w575, "1/TOF", w575, "(1/TOF)^2", w575, "(1/TOF)^3", w575, "Temperature") -> (w581:string)
            }
            frame "Generic BackPoly" {
              n217 = global read "Calib_global.vi" "calib units"() -> (w588:string)
              n218 = for {
                tunnel: w590 -> [w598] mode=indexing
                tunnel: [w596] -> w589 mode=indexing
                n219 = Unbundle By Name(w598) -> ("t/f"=w597:bool)
                n220 = Select(t="NaN not included", s=w597, f="") -> (s? t:f=w596:string)
              }
              n221 = Concatenate Strings(w588, "\t", "Voltage") -> (w591:string)
            }
            frame "Fast FID" {
              w599 = "\t"
              n222 = for {
                tunnel: w605 -> [w612] mode=indexing
                tunnel: [w610] -> w604 mode=indexing
                n223 = Unbundle By Name(w612) -> ("t/f"=w611:bool)
                n224 = Select(t="NaN not included", s=w611, f="") -> (s? t:f=w610:string)
              }
              n225 = Concatenate Strings("Concentration (ppm)" ("Substring"), w599, "Voltage", w599, "Stand dev" ("string"), w599, "ppm/%Density" ("string"), w599, "Temperature" ("string")) -> (w606:string)
            }
            frame "Thermocouple" {
              n226 = for {
                tunnel: w615 -> [w623] mode=indexing
                tunnel: [w621] -> w614 mode=indexing
                n227 = Unbundle By Name(w623) -> ("t/f"=w622:bool)
                n228 = Select(t="NaN not included", s=w622, f="") -> (s? t:f=w621:string)
              }
              n229 = Concatenate Strings("Temperature", "\t", "Voltage") -> (w616:string)
            }
            frame "Cold wire" {
              n230 = for {
                tunnel: w626 -> [w634] mode=indexing
                tunnel: [w632] -> w625 mode=indexing
                n231 = Unbundle By Name(w634) -> ("t/f"=w633:bool)
                n232 = Select(t="NaN not included", s=w633, f="") -> (s? t:f=w632:string)
              }
              n233 = Concatenate Strings("Temperature", "\t", "Voltage") -> (w627:string)
            }
          }
          n234 = Number To Exponential String(number=w485, precision (6)=i16 10) -> (E-format string=w484:string[][])  [unwired: 2 out]
          n235 = Build Array (concatenate)(w484, w483) -> (w482:string[][])
          n236 = Transpose 2D Array(2D array=w482) -> (transposed array=w481:string[][])
          n237 = call "2D_array_to_string.vi"("2D data array"=w481, "Column titles  (separated by tabs)"=w489, "Array title"="Calib points label") -> ("Output string"=w488:string)
        }
        frame #5 {
          n238 = case shown="\"Cross wire angle\"" w635 {
            tunnel: [w643 w650] -> w636
            tunnel: w637 -> [w642 w650]
            frame "Cross wire angle" {
              w641 = "\r\n"
              w647 = "Voltage"
              w648 = "\t"
              n239 = global read "Calib_global.vi" "orig vel calib points"() -> (w638:dbl[][])
              n240 = Concatenate Strings("Velocity (m/s)", w648, w647, w648, w647) -> (w645:string)
              n241 = Number To Exponential String(number=w638, precision (6)=10) -> (E-format string=w640:string[][])  [unwired: 2 out]
              n242 = call "2D_array_to_string.vi"("2D data array"=w640, "Column titles  (separated by tabs)"=w645, "Array title"="Original vel calib points") -> ("Output string"=w644:string)
              n243 = Concatenate Strings(w641, w642, w641, w641, w644) -> (w643:string)
            }
            frame "Generic Linear", Default {
            }
          }
        }
        frame #6 {
          n244 = global read "Calib_global.vi" "aux calib file string"() -> (w660:string)
          n245 = call "Add_label_to_string.vi"("String to write"=w660, "File Label"="Auxiliary constants") -> ("Output string"=w663:string)
          n246 = global read "Calib_global.vi" "Instument setup Info"() -> (w652:string)
          n247 = Concatenate Strings(w658, w657, w656, w652, w653, w654) -> (w655:string)
          n248 = case shown="\"Pulsed Wire\"" w659 {
            tunnel: [w665 w674 w679 w685 w697 w702 w707 w718 w728 w739 w744 w749] -> w661
            tunnel: w663 -> [_ _ _ w684 w692 _ _ _ _ _ _ _]
            tunnel: " calib label" -> [w668 w671 w676 _ _ w699 w704 w715 w725 w736 w741 w746]
            tunnel: w655 -> [w667 w670 w675 w681 w690 w698 w703 w710 w724 w733 w740 w745]
            tunnel: "\r\n" -> [_ _ _ w680 w689 _ _ _ _ _ _ _]
            frame "Propeller anemometer" {
              n249 = Concatenate Strings("Prop", w668) -> (w666:string)
              n250 = call "Add_label_to_string.vi"("String to write"=w667, "File Label"=w666) -> ("Output string"=w665:string)
            }
            frame "Pressure Transducer" {
              n251 = Concatenate Strings("Mano", w671) -> (w672:string)
              n252 = call "Add_label_to_string.vi"("String to write"=w670, "File Label"=w672) -> ("Output string"=w674:string)
            }
            frame "Hot wire" {
              n253 = Concatenate Strings("HW", w676) -> (w678:string)
              n254 = call "Add_label_to_string.vi"("String to write"=w675, "File Label"=w678) -> ("Output string"=w679:string)
            }
            frame "Cross wire velocity" {
              n255 = global read "Calib_global.vi" "Angle/vel calib file string"() -> (w682:string)
              n256 = call "Add_label_to_string.vi"("String to write"=w681, "File Label"="Cross wire velocity calib label") -> ("Output string"=w686:string)
              n257 = call "Add_label_to_string.vi"("String to write"=w682, "File Label"="Cross wire angle calib label") -> ("Output string"=w683:string)
              n258 = Concatenate Strings(w686, w680, w684, w680, w680, w683) -> (w685:string)
            }
            frame "Cross wire angle" {
              n259 = global read "Calib_global.vi" "Angle/vel calib file string"() -> (w691:string)
              n260 = call "Add_label_to_string.vi"("String to write"=w691, "File Label"="Cross wire velocity calib label") -> ("Output string"=w694:string)
              n261 = call "Add_label_to_string.vi"("String to write"=w690, "File Label"="Cross wire angle calib label") -> ("Output string"=w693:string)
              n262 = Concatenate Strings(w694, w689, w692, w689, w689, w693) -> (w697:string)
            }
            frame "Generic Linear" {
              n263 = Concatenate Strings("Generic Inst", w699) -> (w700:string)
              n264 = call "Add_label_to_string.vi"("String to write"=w698, "File Label"=w700) -> ("Output string"=w702:string)
            }
            frame "Generic Polynomial" {
              n265 = Concatenate Strings("Generic Polynomial", w704) -> (w705:string)
              n266 = call "Add_label_to_string.vi"("String to write"=w703, "File Label"=w705) -> ("Output string"=w707:string)
            }
            frame "Pulsed Wire" {
              n267 = global read "PWAtasksGLOBAL.vi" "PWA Lookup Table"() -> (w714:dbl[])
              n268 = for {
                tunnel: w714 -> [w723] mode=indexing
                shift-right: [w719] -> w712
                shift-left: "" -> [w720]
                n269 = Number To Exponential String(number=w723) -> (E-format string=w721:string)  [unwired: 3 out]
                n270 = Concatenate Strings(w720, w721, "\r\n") -> (w719:string)
              }
              n271 = Concatenate Strings("Pulsed wire", w715) -> (w716:string)
              n272 = call "Add_label_to_string.vi"("String to write"=w712, "File Label"="Pulsed_wire_lookup_table") -> ("Output string"=w709:string)
              n273 = Concatenate Strings(w710, w709) -> (w708:string)
              n274 = call "Add_label_to_string.vi"("String to write"=w708, "File Label"=w716) -> ("Output string"=w718:string)
            }
            frame "Generic BackPoly" {
              n275 = Concatenate Strings("Generic BackPoly", w725) -> (w726:string)
              n276 = call "Add_label_to_string.vi"("String to write"=w724, "File Label"=w726) -> ("Output string"=w728:string)
            }
            frame "Fast FID" {
              n277 = Concatenate Strings("Fast FID", w736) -> (w737:string)
              n278 = call "Replace_data_in_setup_string.vi"("New data string"="0.00", "Input string"=w733, "Variable name"="Fast FID Bkgnd") -> ("Appended string"=w730:string)
              n279 = call "Replace_data_in_setup_string.vi"("New data string"="0.00", "Input string"=w730, "Variable name"="Fast FID Bkgnd Variance") -> ("Appended string"=w729:string)
              n280 = call "Add_label_to_string.vi"("String to write"=w729, "File Label"=w737) -> ("Output string"=w739:string)
            }
            frame "Thermocouple" {
              n281 = Concatenate Strings("Thermocouple", w741) -> (w742:string)
              n282 = call "Add_label_to_string.vi"("String to write"=w740, "File Label"=w742) -> ("Output string"=w744:string)
            }
            frame "Cold wire" {
              n283 = Concatenate Strings("Cold wire", w746) -> (w747:string)
              n284 = call "Add_label_to_string.vi"("String to write"=w745, "File Label"=w747) -> ("Output string"=w749:string)
            }
          }
          n285 = global write "Calib_global.vi" "Header string"(w661) -> ()
        }
      }
    }
    frame #5 {
      n286 = local read "Point selector 4"() -> (→"Point selector 4 out":T1)
      n287 = local read "Point selector 3"() -> (→"Point selector 3 out":cluster{"Y":dbl, "X":dbl, "t/f":bool}[])
    }
  }
